vi "Lector_Audio.vi"(11 "path":path) -> (0 "Error_B":errorcluster, 1 "task ID out":T1 format="%.0x", 2 "Error_A":errorcluster, 3 "sound file refnum out":T2)   [LabVIEW 2017]
uses:
  <vilib>/sound2/lvsound2.llb/Sound File Refnum.ctl
  <vilib>/sound2/lvsound2.llb/Sound Output Task ID.ctl
  <vilib>/sound2/lvsound2.llb/Sampling Mode.ctl
  <vilib>/sound2/lvsound2.llb/Sound File Read Open.vi
  <vilib>/sound2/lvsound2.llb/Sound File Info (refnum).vi
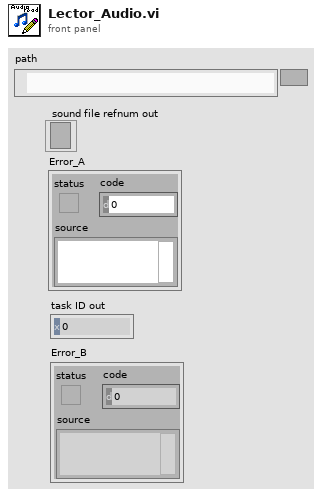
[diagram p1: front panel]
types:
  T1 = typedef "Sound Output Task ID.ctl" = u32
  T2 = typedef "Sound File Refnum.ctl" = refnum<file>
  T3 = typedef "Sampling Mode.ctl" = i32
  T4 = typedef "Sound Data Format.ctl" = cluster{"sample rate (S/s)":dbl, "number of channels":i32, "bits per sample":i32}
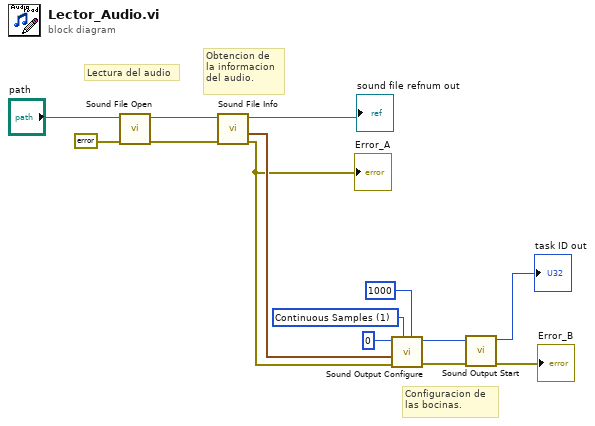
[diagram p0: block diagram]
diagram:
  w8 = T3 1 items=["Finite Samples", "Continuous Samples"] ("sample mode")
  # "Obtencion de\nla informacion\ndel audio."
  # "Lectura del audio"
  # "Configuracion de\nlas bocinas."
  n1 = call-poly <vilib>:"Sound File Open.vi"("error in (no error)"=errorcluster {"status"=FALSE, "code"=0, "source"=""}, "path"="path") -> ("error out"=w11:errorcluster, "sound file refnum"=w10:T2)  [unwired: 8 in]
  n2 = call-poly <vilib>:"Sound File Info.vi"("error in (no error)"=w11, "sound file refnum"=w10) -> ("error out"=w5:errorcluster, "sound format"=w6:T4, "sound file refnum out"=→"sound file refnum out":T2)  [unwired: 6 in, 1 out]
  "Error_A" <- w5
  n3 = call <vilib>:"Sound Output Configure.vi"("number of samples/ch"=1000, "sample mode"=w8, "error in (no error)"=w5, "sound format"=w6, "device ID"=u32 0) -> ("error out"=w13:errorcluster, "task ID"=w14:T1)  [unwired: 5 in]
  n4 = call <vilib>:"Sound Output Start.vi"("error in (no error)"=w13, "task ID"=w14) -> ("error out"=→"Error_B":errorcluster, "task ID out"=→"task ID out":T1)  [unwired: 8 in]
